vi "NISE.remote.Property is Enum.vi"(0 "SLSC Remote in":refnum<class "SLSC Interface.lvclass">, 5 "property":refnum<k21>, 11 "error in (no error)":errorcluster) -> (4 "SLSC Remote out":refnum<class "SLSC Interface.lvclass">, 6 "property out":refnum<k21>, 10 "Prop.IsEnum":bool, 15 "error out":errorcluster)   [LabVIEW 2016, in "SLSC Interface.lvclass"]
uses:
  SLSC Interface Class/SLSC Interface.lvclass
  SLSC Interface Class/SLSC Interface.lvclass/SLSC Interface.ctl
  SLSC Interface Class/NISE.Read client handle.vi
  SLSC Interface Class/NISE.Read URL.vi
  SLSC Interface Class/NISE.Read session.vi
  <vilib>/NI/NI JSONRPC Server Framework/Classes/Server/server.Format Client Request (Auto-Increment).vi
  <vilib>/httpClient/POSTBuffer.vi
  <vilib>/httpClient/LabVIEWHTTPClient.lvlib
  <vilib>/NI/NI JSONRPC Server Framework/Classes/Server/JSONRPC Server.lvclass
  <vilib>/NI/JSON Support for LabVIEW/JSON Value/JSON Value.lvclass
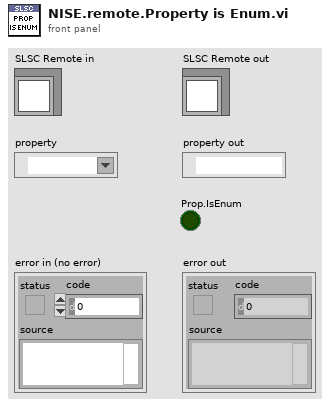
[diagram p1: front panel]
types:
  T1 = typedef "LabVIEWHTTPClient.lvlib/ClientHandle.ctl" = refnum<k1>
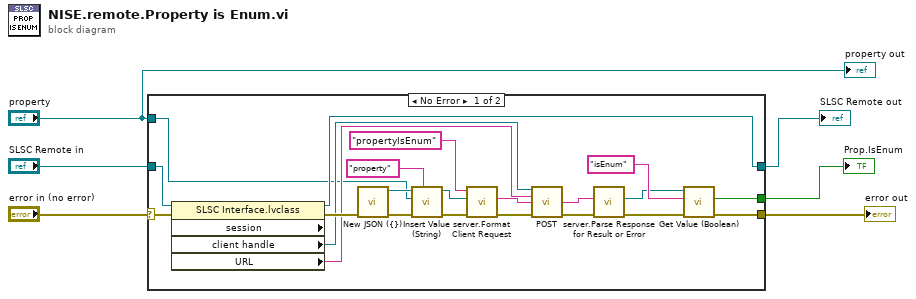
[diagram p0: block diagram]
diagram:
  n1 = case shown="No Error" "error in (no error)" {
    selector: "error in (no error)" -> [w26 w29]
    tunnel: "property" -> [w9 _]
    tunnel: "SLSC Remote in" -> [w28 w30]
    tunnel: [w27 w30] -> w3
    tunnel: [w14 w29] -> w4
    tunnel: [w11 _] -> w2
    frame No Error {
      n2 = property class="SLSC Interface.lvclass" props=["session", "client handle", "URL"](reference=w28, error in=w26) -> (reference out=w27:refnum<class "SLSC Interface.lvclass">, error out=w25:errorcluster, "client handle"=w19:T1, "URL"=w18:string)  [unwired: 1 out]
      n3 = call <vilib>:"New JSON ({}).vi"("error in (no error)"=w25) -> ("error out"=w24:errorcluster, "JSON Value out"=w10:refnum<class "JSON Value.lvclass">)  [unwired: 9 in]
      n4 = call <vilib>:"Insert Value (String).vi"("key"="property" ("Name"), "error in (no error)"=w24, "value"=w9, "JSON Value in"=w10) -> ("error out"=w23:errorcluster, "JSON Value out"=w20:refnum<class "JSON Value.lvclass">)  [unwired: 5 in, 1 out]
      n5 = call-poly <vilib>:"server.Format Client Request.vi"("error in (no error)"=w23, "JSON Value in"=w20, "method"="propertyIsEnum") -> ("error out"=w17:errorcluster, "Request String"=w21:string)  [unwired: 7 in]
      n6 = call-poly <vilib>:"POST.vi"("client handle"=w19, "url"=w18, "buffer"=w21, "error in (no error)"=w17) -> ("body"=w16:string, "error out"=w15:errorcluster)  [unwired: 8 in, 2 out]
      n7 = call <vilib>:"server.Parse Response for Result or Error.vi"("error in"=w15, "Response String In"=w16) -> ("error out"=w12:errorcluster, "JSON Value out"=w7:refnum<class "JSON Value.lvclass">)  [unwired: 7 in, 1 out]
      n8 = call <vilib>:"Get Value (Boolean).vi"("error in (no error)"=w12, "key"="isEnum" ("Parameter Name"), "JSON Value in"=w7) -> ("error out"=w14:errorcluster, "value"=w11:bool)  [unwired: 7 in]
    }
    frame Error {
    }
  }
  "error out" <- w4
  "SLSC Remote out" <- w3
  "Prop.IsEnum" <- w2
  "property out" <- "property"
